vi "Add point to Route.vi"(8 "Error In":errorcluster, 10 "New Point":refnum<k24>, 11 "Route Index":i32) -> (0 "Error Out":errorcluster)   [LabVIEW 2014]
uses:
  C:/Robotic Systems/Products/AgFalcon/Software/Ground Station/Data/Mapping DLL/GMap.NET.Core.dll
  Data/Mapping DLL/GMap.NET.Core.dll
  C:/Robotic Systems/Products/AgFalcon/Software/Ground Station/Data/Mapping DLL/GMap.NET.WindowsForms.dll
  Data/Mapping DLL/GMap.NET.WindowsForms.dll
  Reference/SubVI/GMap DLL Refernce.vi
  Reference/SubVI/Main Map Control Refernce.vi
  Missions/FGVs/Currently Selected Virtual WP/Methods/Set Current Virtual Waypoint.vi
  Application Support/Data Processing Queue/SubVI/Set Operations Queue.vi
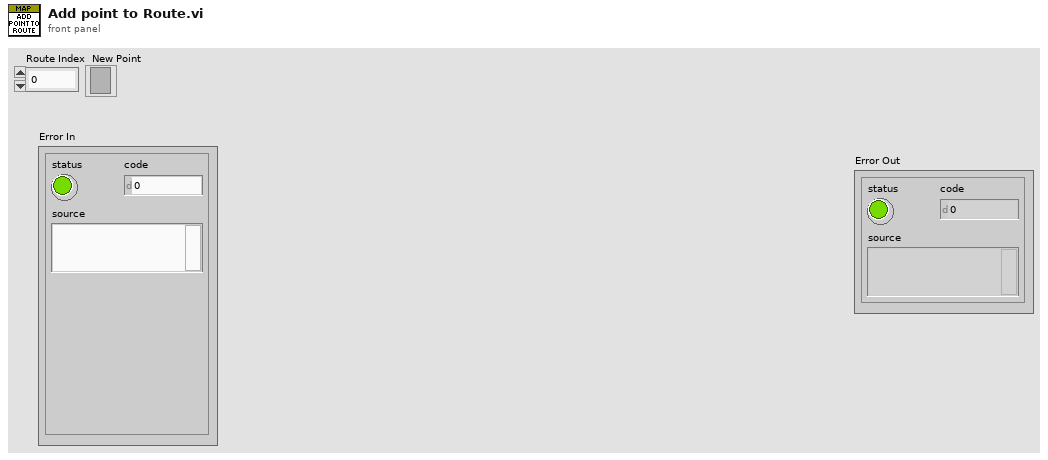
[diagram p1: front panel]
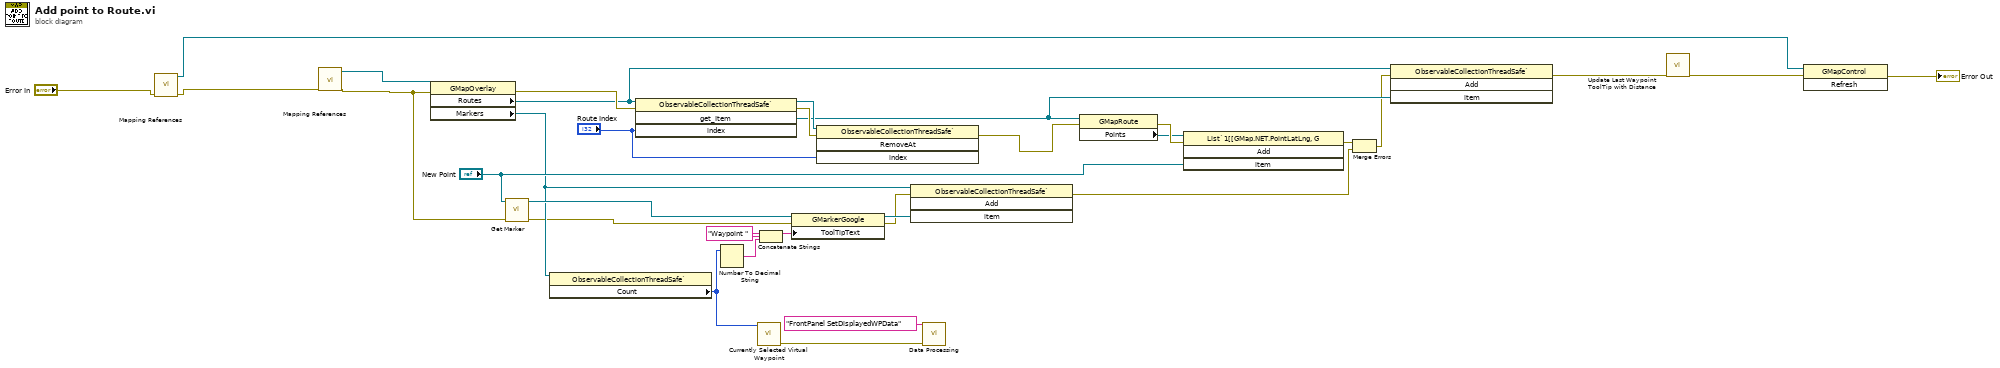
[diagram p0: block diagram]
diagram:
  n1 = call-poly "Mapping References.vi"("Error In"="Error In") -> ("Error Out"=w23:errorcluster, "GMap DLL Reference"=w21:refnum<k24>)  [unwired: 9 in]
  n2 = call-poly "Mapping References.vi"("Error In"=w23) -> ("Error Out"=w19:errorcluster, "Main Map Reference"=w24:refnum<k24>)  [unwired: 9 in]
  n3 = property class="GMapOverlay"(reference=w24, error in=w19) -> (error out=w32:errorcluster, "Routes"=w25:refnum<k24>, "Markers"=w12:refnum<k24>)  [unwired: 1 out]
  n4 = call "Get Marker.vi"("Error In"=w19, "Point"="New Point") -> ("error out"=w8:errorcluster, "new reference"=w15:refnum<k24>)  [unwired: 8 in]
  n5 = property class="ObservableCollectionThreadSafe`"(reference=w12) -> ("Count"=w5:i32)  [unwired: 1 in, 2 out]
  n6 = invoke class="ObservableCollectionThreadSafe`" method="get_Item"(reference=w25, error in=w32, "index"="Route Index") -> (reference out=w30:refnum<k24>, error out=w31:errorcluster, "get_Item"=w27:refnum<k24>)  [unwired: 1 in, 1 out]
  n7 = Number To Decimal String(number=w5) -> (decimal integer string=w11:string)  [unwired: 1 in]
  n8 = call-poly "Currently Selected Virtual Waypoint.vi"("Waypoint Index In"=w5) -> ("Error Out"=w3:errorcluster)  [unwired: 10 in]
  n9 = Concatenate Strings("Waypoint " ("string"), w11) -> (w9:string)
  n10 = property class="GMarkerGoogle"(reference=w15, error in=w8, "ToolTipText"=w9) -> (reference out=w14:refnum<k24>, error out=w7:errorcluster)
  n11 = invoke class="ObservableCollectionThreadSafe`" method="RemoveAt"(reference=w30, error in=w31, "index"="Route Index") -> (error out=w6:errorcluster)  [unwired: 1 in, 3 out]
  n12 = invoke class="ObservableCollectionThreadSafe`" method="Add"(reference=w12, error in=w7, "item"=w14) -> (error out=w17:errorcluster)  [unwired: 1 in, 3 out]
  n13 = call-poly "Data Processing.vi"("error in (no error)"=w3, "Command"="FrontPanel SetDisplayedWPData") -> ()  [unwired: 9 in, 1 out]
  n14 = property class="GMapRoute"(reference=w27, error in=w6) -> (error out=w29:errorcluster, "Points"=w28:refnum<k24>)  [unwired: 1 out]
  n15 = invoke class="List`1[[GMap.NET.PointLatLng, G" method="Add"(reference=w28, error in=w29, "item"="New Point") -> (error out=w18:errorcluster)  [unwired: 1 in, 3 out]
  n16 = Merge Errors(w18, w17) -> (w16:errorcluster)
  n17 = invoke class="ObservableCollectionThreadSafe`" method="Add"(reference=w25, error in=w16, "item"=w27) -> (error out=w2:errorcluster)  [unwired: 1 in, 3 out]
  n18 = call "Update Last Waypoint ToolTip with Distance.vi"("Error In"=w2) -> ("Error Out"=w1:errorcluster)  [unwired: 10 in]
  n19 = invoke class="GMapControl" method="Refresh"(reference=w21, error in=w1) -> (error out=→"Error Out":errorcluster)  [unwired: 1 in, 2 out]
